vi "g_Joystick1.vi"(7 "Action":enum16{"initialize", "read", "write"}(ring), 9 "Buttons":bool[](array[boolean]), 10 "Axes":dbl[](array[numeric]), 11 "DebounceLength":i32=1) -> (1 "Buttons out":T2, 2 "Axes out":T1 {"Axis 6" format="%#_4g"; "Axis 5" format="%#_4g"; "Axis 4" format="%#_4g"; "Axis 3" format="%#_4g"; "Axis 2" format="%#_4g"; "Axis 1" format="%#_4g"}, 4 "Array":cluster{"DbArray":bool[]}[](array[cluster]))   [LabVIEW 2017]
uses:
  Ctrl Refs/JoyStick1.ctl
  Ctrl Refs/JoyStick1(Analog).ctl
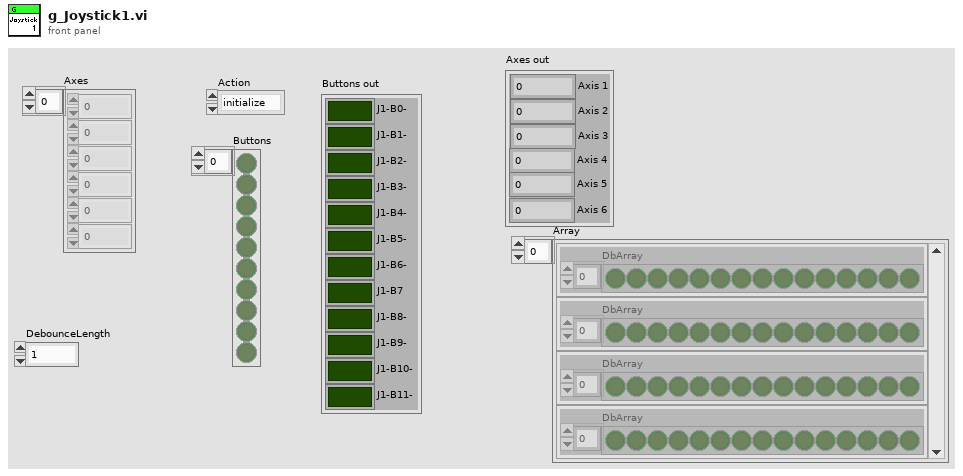
[diagram p1: front panel]
types:
  T1 = typedef "JoyStick1(Analog).ctl" = cluster{"Axis 1":dbl, "Axis 2":dbl, "Axis 3":dbl, "Axis 4":dbl, "Axis 5":dbl, "Axis 6":dbl}
  T2 = typedef "JoyStick1.ctl" = cluster{"J1-B0-":bool, "J1-B1-":bool, "J1-B2-":bool, "J1-B3- ":bool, "J1-B4-":bool, "J1-B5-":bool, "J1-B6-":bool, "J1-B7":bool, "J1-B8-":bool, "J1-B9-":bool, "J1-B10-":bool, "J1-B11-":bool}
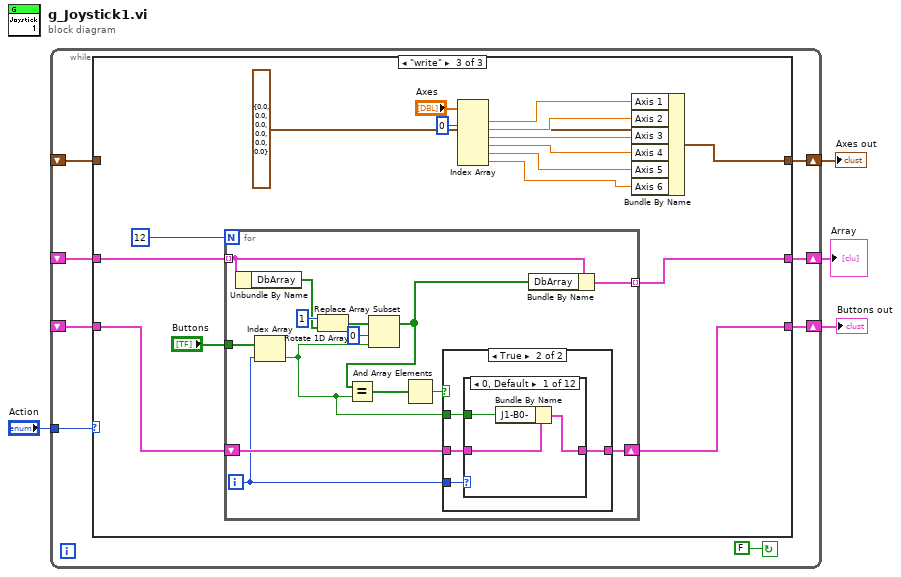
[diagram p0: block diagram]
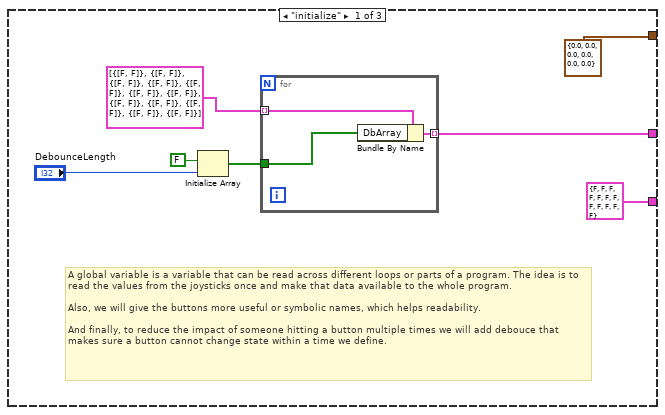
[diagram p2: hidden frame]
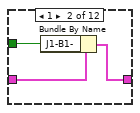
[diagram p5: hidden frame]
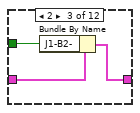
[diagram p6: hidden frame]
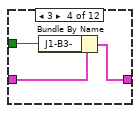
[diagram p7: hidden frame]
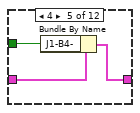
[diagram p8: hidden frame]
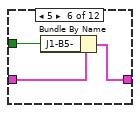
[diagram p9: hidden frame]
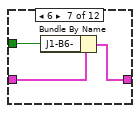
[diagram p10: hidden frame]
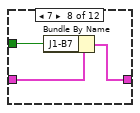
[diagram p11: hidden frame]
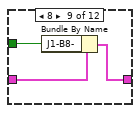
[diagram p12: hidden frame]
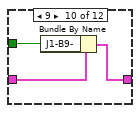
[diagram p13: hidden frame]
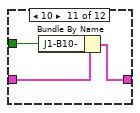
[diagram p14: hidden frame]
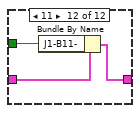
[diagram p15: hidden frame]
diagram:
  n1 = while {
    tunnel: "Action" -> [w11]
    shift-right: [w10] -> w2
    shift-left: _ -> [w9]
    shift-right: [w8] -> w3
    shift-left: _ -> [w7]
    shift-right: [w6] -> w1
    shift-left: _ -> [w5]
    stop <- FALSE continue-if-true
    n2 = case shown="\"write\"" w11 {
      tunnel: [T1 {"Axis 1"=0.0, "Axis 2"=0.0, "Axis 3"=0.0, "Axis 4"=0.0, "Axis 5"=0.0, "Axis 6"=0.0} ("Axes out") w25 w37] -> w10
      tunnel: w9 -> [_ w25 _]
      tunnel: [w15 w24 w33] -> w8
      tunnel: w7 -> [_ w24 w34]
      tunnel: [T2 {"J1-B0-"=FALSE, "J1-B1-"=FALSE, "J1-B2-"=FALSE, "J1-B3- "=FALSE, "J1-B4-"=FALSE, "J1-B5-"=FALSE, "J1-B6-"=FALSE, "J1-B7"=FALSE, "J1-B8-"=FALSE, "J1-B9-"=FALSE, "J1-B10-"=FALSE, "J1-B11-"=FALSE} ("Buttons out") w23 w31] -> w6
      tunnel: w5 -> [_ w23 w32]
      frame "initialize" {
        # "A global variable is a variable that can be read across different loops or parts of a program. The idea is to read the values from the joysticks once and make that data available to the whole program.\n \nAlso, we will give the buttons more useful or symbolic names, which helps readability. \n\nAnd finally, to reduce the impact of someone hitting a button multiple times we will add debouce that makes sure a button cannot change state within a time we define."
        n3 = Initialize Array(FALSE, "DebounceLength") -> (w16:bool[])
        n4 = for {
          tunnel: cluster{"DbArray":bool[]}[] [{"DbArray"=[FALSE, FALSE]}, {"DbArray"=[FALSE, FALSE]}, {"DbArray"=[FALSE, FALSE]}, {"DbArray"=[FALSE, FALSE]}, {"DbArray"=[FALSE, FALSE]}, {"DbArray"=[FALSE, FALSE]}, {"DbArray"=[FALSE, FALSE]}, {"DbArray"=[FALSE, FALSE]}, {"DbArray"=[FALSE, FALSE]}, {"DbArray"=[FALSE, FALSE]}, {"DbArray"=[FALSE, FALSE]}, {"DbArray"=[FALSE, FALSE]}] -> [w22] mode=indexing
          tunnel: w16 -> [w21]
          tunnel: [w20] -> w15 mode=indexing
          n5 = Bundle By Name(cluster=w22, "DbArray"=w21) -> (w20:cluster{"DbArray":bool[]})
        }
      }
      frame "read", Default {
      }
      frame "write" {
        n6 = for {
          N: 12 -> [_]
          tunnel: "Buttons" -> [w44]
          tunnel: w34 -> [w55] mode=indexing
          tunnel: [w51] -> w33 mode=indexing
          shift-right: [w49] -> w31
          shift-left: w32 -> [w50]
          i -> [w42]
          n7 = Unbundle By Name(w55) -> ("DbArray"=w48:bool[])
          n8 = Index Array(array=w44, index=w42) -> (element=w43:bool)
          n9 = Rotate 1D Array(1:w48, 2:1 ("n")) -> (0:w53:bool[])
          n10 = Replace Array Subset(array=w53, new element=w43, index=0) -> (w47:bool[])
          n11 = Equal?(x=w47, y=w43) -> (x = y?=w46:bool[])
          n12 = And Array Elements(Boolean array=w46) -> (logical AND=w45:bool)
          n13 = case shown="True" w45 {
            tunnel: w42 -> [_ w60]
            tunnel: w50 -> [w56 w59]
            tunnel: [w56 w58] -> w49
            tunnel: w43 -> [_ w57]
            frame False {
            }
            frame True {
              n14 = case shown="0, Default" w60 {
                tunnel: w59 -> [w63 w66 w69 w72 w75 w78 w81 w84 w87 w90 w93 w96]
                tunnel: [w62 w65 w68 w71 w74 w77 w80 w83 w86 w89 w92 w95] -> w58
                tunnel: w57 -> [w61 w64 w67 w70 w73 w76 w79 w82 w85 w88 w91 w94]
                frame 0, Default {
                  n15 = Bundle By Name(cluster=w63, "J1-B0-"=w61) -> (w62:T2)
                }
                frame 1 {
                  n16 = Bundle By Name(cluster=w66, "J1-B1-"=w64) -> (w65:T2)
                }
                frame 2 {
                  n17 = Bundle By Name(cluster=w69, "J1-B2-"=w67) -> (w68:T2)
                }
                frame 3 {
                  n18 = Bundle By Name(cluster=w72, "J1-B3-"=w70) -> (w71:T2)
                }
                frame 4 {
                  n19 = Bundle By Name(cluster=w75, "J1-B4-"=w73) -> (w74:T2)
                }
                frame 5 {
                  n20 = Bundle By Name(cluster=w78, "J1-B5-"=w76) -> (w77:T2)
                }
                frame 6 {
                  n21 = Bundle By Name(cluster=w81, "J1-B6-"=w79) -> (w80:T2)
                }
                frame 7 {
                  n22 = Bundle By Name(cluster=w84, "J1-B7"=w82) -> (w83:T2)
                }
                frame 8 {
                  n23 = Bundle By Name(cluster=w87, "J1-B8-"=w85) -> (w86:T2)
                }
                frame 9 {
                  n24 = Bundle By Name(cluster=w90, "J1-B9-"=w88) -> (w89:T2)
                }
                frame 10 {
                  n25 = Bundle By Name(cluster=w93, "J1-B10-"=w91) -> (w92:T2)
                }
                frame 11 {
                  n26 = Bundle By Name(cluster=w96, "J1-B11-"=w94) -> (w95:T2)
                }
              }
            }
          }
          n27 = Bundle By Name(cluster=w55, "DbArray"=w47) -> (w51:cluster{"DbArray":bool[]})
        }
        n28 = Index Array(array="Axes", index #1=0 ("index")) -> (element #1=w40:dbl, element #2=w39:dbl, element #3=w38:dbl, element #4=w28:dbl, element #5=w27:dbl, element #6=w26:dbl)  [unwired: 5 in]
        n29 = Bundle By Name(cluster=T1 {"Axis 1"=0.0, "Axis 2"=0.0, "Axis 3"=0.0, "Axis 4"=0.0, "Axis 5"=0.0, "Axis 6"=0.0} ("Axes out"), "Axis 1"=w40, "Axis 2"=w39, "Axis 3"=w38, "Axis 4"=w28, "Axis 5"=w27, "Axis 6"=w26) -> (w37:T1)
      }
    }
  }
  "Buttons out" <- w1
  "Axes out" <- w2
  "Array" <- w3
